vi "Theta Align Type.vi"(10 "Robot Pose":cluster{"X":dbl, "Y":dbl}, 11 "Type":enum16{"Hub", "Corner of Field"}(ring)) -> (2 "Blue Alliance?":bool, 3 "Setpoint Pose":cluster{"X":dbl, "Y":dbl})   [LabVIEW 2025]
uses:
  <vilib>/Rock Robotics/WPI/DriverStation/WPI_DriverStationAllianceInfo.ctl
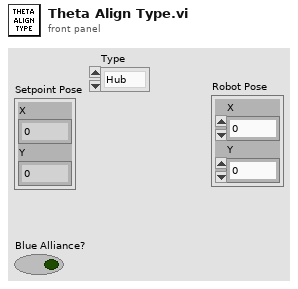
[diagram p1: front panel]
types:
  T1 = typedef "WPI_DriverStationAllianceInfo.ctl" = enum16{"Red", "Blue", "Invalid"}
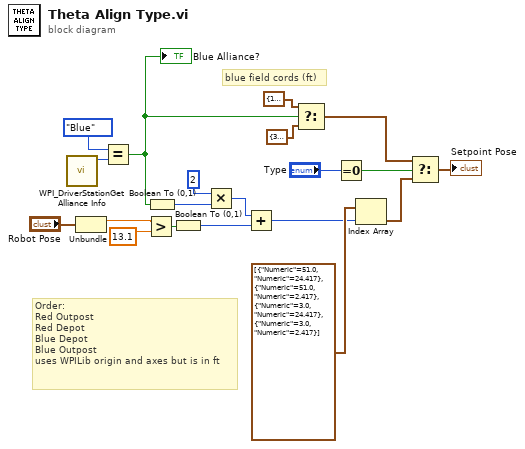
[diagram p0: block diagram]
diagram:
  # "Order:\nRed Outpost\nRed Depot\nBlue Depot\nBlue Outpost\nuses WPILib origin and axes but is in ft"
  # "blue field cords (ft)"
  n1 = call <vilib>:"WPI_DriverStationGet Alliance Info.vi"() -> ("Alliance"=w18:T1)  [unwired: 6 in, 5 out]
  n2 = Unbundle("Robot Pose") -> ("X"=w15:dbl)  [unwired: 1 out]
  n3 = Equal?(x=WPI_DriverStationAllianceInfo."Blue", y=w18) -> (x = y?=w11:bool)
  "Blue Alliance?" <- w11
  n4 = Greater?(x=w15, y=13.1) -> (0:w13:bool)
  n5 = Boolean To (0,1)(Boolean=w11) -> (0, 1=w1:i16)
  n6 = Boolean To (0,1)(Boolean=w13) -> (0, 1=w2:i16)
  n7 = Multiply(x=i16 2, y=w1) -> (x*y=w3:i16)
  n8 = Add(x=w3, y=w2) -> (x+y=w5:i16)
  n9 = Select(t=cluster{"Numeric":dbl, "Numeric":dbl} {"Numeric"=15.31, "Numeric"=13.19333} ("x"), s=w11, f=cluster{"Numeric":dbl, "Numeric":dbl} {"Numeric"=39.04667, "Numeric"=13.19333} ("x")) -> (s? t:f=w8:cluster{"Numeric":dbl, "Numeric":dbl})
  n10 = Equal To 0?(x="Type") -> (x = 0?=w9:bool)
  n11 = Index Array(array=cluster{"Numeric":dbl, "Numeric":dbl}[] [{"Numeric"=51.0, "Numeric"=24.417}, {"Numeric"=51.0, "Numeric"=2.417}, {"Numeric"=3.0, "Numeric"=24.417}, {"Numeric"=3.0, "Numeric"=2.417}] ("x"), index=w5) -> (element=w7:cluster{"Numeric":dbl, "Numeric":dbl})
  n12 = Select(t=w8, s=w9, f=w7) -> (s? t:f=→"Setpoint Pose":cluster{"Numeric":dbl, "Numeric":dbl})
